vi "Write File Name.vi"(8 "error in (no error)":errorcluster, 10 "File Name":string, 11 "Setup File in":refnum<class "Setup File.lvclass">) -> (0 "error out":errorcluster, 3 "Setup File out":refnum<class "Setup File.lvclass">)   [LabVIEW 2018, in "Setup File.lvclass"]
doc: "Este VI escreve o nome do arquivo na classe."
uses:
  Setup File.lvclass
  Setup File.lvclass/Setup File.ctl
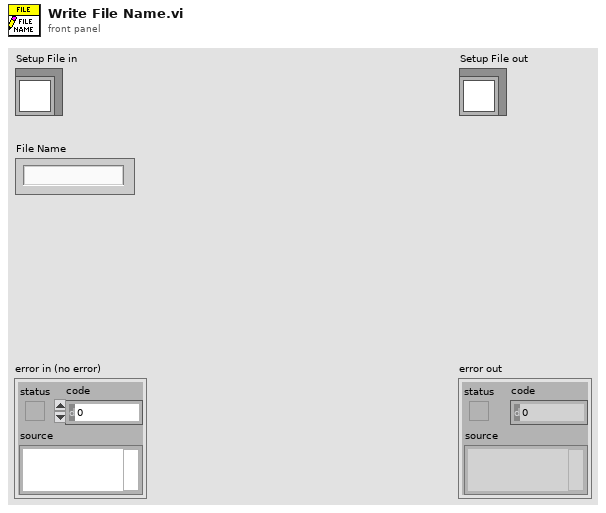
[diagram p1: front panel]
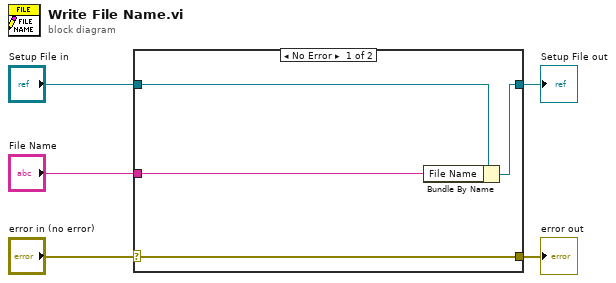
[diagram p0: block diagram]
diagram:
  n1 = case shown="No Error" "error in (no error)" {
    selector: "error in (no error)" -> [w9 w10]
    tunnel: [w9 w10] -> w4
    tunnel: [w7 w11] -> w2
    tunnel: "Setup File in" -> [w8 w11]
    tunnel: "File Name" -> [w6 _]
    frame No Error {
      n2 = Bundle By Name(cluster=w8, "File Name"=w6) -> (w7:refnum<class "Setup File.lvclass">)
    }
    frame Error {
    }
  }
  "error out" <- w4
  "Setup File out" <- w2
